vi "Write Rename.vi"(8 "error in (no error)":errorcluster, 10 "Rename":string, 11 "_Rename in":refnum<class "_Rename.lvclass">) -> (0 "error out":errorcluster, 3 "_Rename out":refnum<class "_Rename.lvclass">)   [LabVIEW 2021, in "_Rename.lvlib" / "_Rename.lvclass"]
uses:
  _Rename.lvclass
  _Rename.lvclass/_Rename.ctl
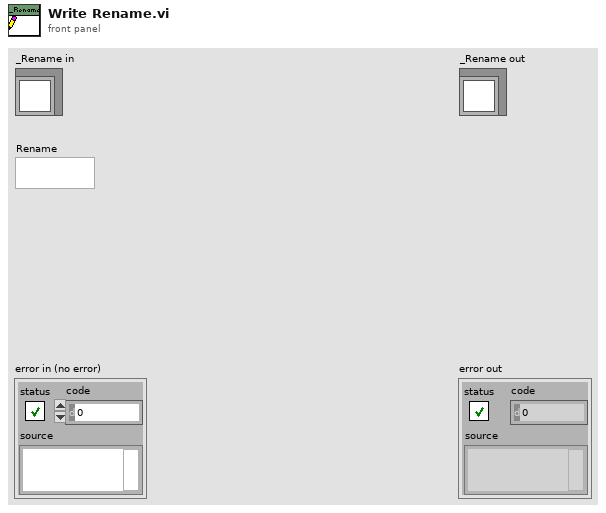
[diagram p1: front panel]
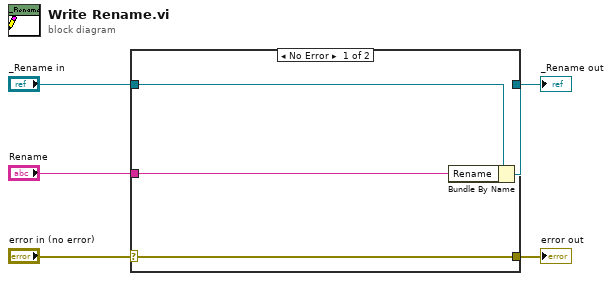
[diagram p0: block diagram]
diagram:
  n1 = case shown="No Error" "error in (no error)" {
    selector: "error in (no error)" -> [w9 w10]
    tunnel: [w9 w10] -> w4
    tunnel: [w7 w11] -> w2
    tunnel: "_Rename in" -> [w8 w11]
    tunnel: "Rename" -> [w6 _]
    frame No Error {
      n2 = Bundle By Name(cluster=w8, "Rename"=w6) -> (w7:refnum<class "_Rename.lvclass">)
    }
    frame Error {
    }
  }
  "error out" <- w4
  "_Rename out" <- w2
